vi "Add BaseNodeType Child.vi"(8 "error in":errorcluster, 10 "child BaseNodeType in":refnum<k24>, 11 "parent ref in":T1 format="%.0x") -> (0 "error out":errorcluster, 1 "child ref":T1 format="%.0x", 2 "child BaseNodeType out":refnum<k24>, 3 "parent ref out":T1 format="%.0x")   [LabVIEW 2017, in "Import Export.lvlib"]
uses:
  Import Export.lvlib
  NationalInstruments.VeriStand.SystemStorage
  <vilib>/NI Veristand/Custom Device API/Custom Device Item Ref.ctl
  System Explorer Action.ctl
  <vilib>/NI VeriStand/Custom Device API/Custom Device API.lvlib
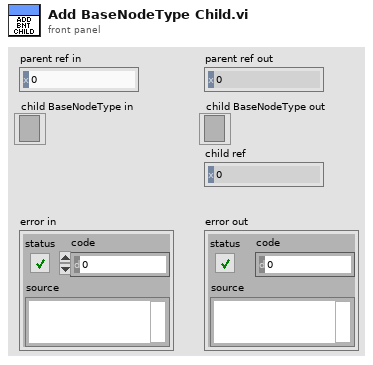
[diagram p1: front panel]
types:
  T1 = typedef "Custom Device API.lvlib/Custom Device Item Ref.ctl" = u64
  T2 = typedef "Import Export.lvlib/System Explorer Action.ctl" = u16
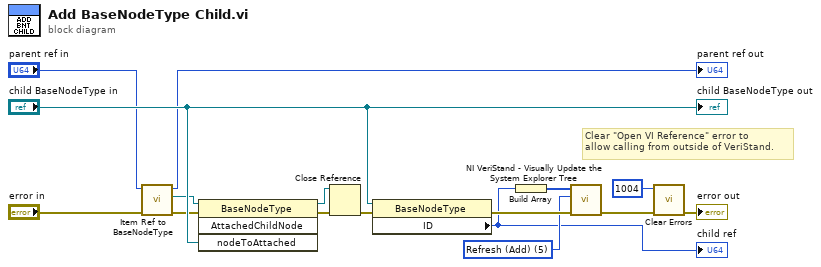
[diagram p0: block diagram]
diagram:
  w6 = T2 5 items=["Refresh (Add)"=5, "Refresh (Repopulate node)"=7, "Refresh (Delete)"=9] ("Action")
  # "Clear \"Open VI Reference\" error to\nallow calling from outside of VeriStand."
  n1 = call "Item Ref to BaseNodeType.vi"("error in (no error)"="error in", "item ref in"="parent ref in") -> ("error out"=w14:errorcluster, "BaseNodeType"=w12:refnum<k24>, "item ref out"=→"parent ref out":T1)  [unwired: 7 in]
  n2 = invoke class="BaseNodeType" method="AttachedChildNode"(reference=w12, error in=w14, "nodeToAttached"="child BaseNodeType in") -> (reference out=w4:refnum<k24>, error out=w7:errorcluster)  [unwired: 1 in, 2 out]
  n3 = Close Reference(reference=w4, error in (no error)=w7) -> (error out=w11:errorcluster)
  n4 = property class="BaseNodeType"(reference="child BaseNodeType in", error in=w11) -> (error out=w15:errorcluster, "ID"=w1:u64)  [unwired: 1 out]
  "child ref" <- w1
  n5 = Build Array(w1) -> (w5:u64[])
  n6 = call "NI VeriStand - Visually Update the System Explorer Tree.vi"("error in (no error)"=w15, "Action"=w6, "Node IDs"=w5) -> ("error out"=w9:errorcluster)  [unwired: 8 in]
  n7 = call <vilib>:"Clear Errors.vi"("error in (no error)"=w9, "specific error code to clear (0: all)"=1004) -> ("error out"=→"error out":errorcluster)  [unwired: 4 in, 1 out]
  "child BaseNodeType out" <- "child BaseNodeType in"
